vi "map.get.vi"(11 "CLZ Comics in":refnum<class "CLZ Comics.lvclass">) -> (2 "map":map{i32, T1}(c390), 3 "CLZ Comics out":refnum<class "CLZ Comics.lvclass">)   [LabVIEW 2024, in "CLZ_to_ComicVine.lvlib" / "CLZ Comics.lvclass"]
uses:
  CLZ Comics.lvclass
  CLZ Comics.lvclass/CLZ Comics.ctl
  typedefs/issue_number--cluster.ctl
  typedefs/volume--cluster.ctl
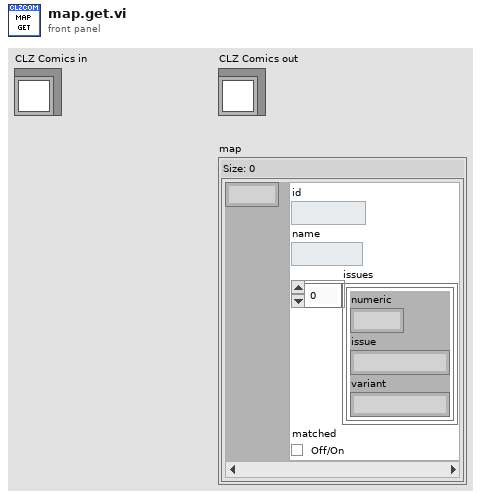
[diagram p1: front panel]
types:
  T1 = typedef "CLZ_to_ComicVine.lvlib/CLZ Comics.lvclass/volume--cluster.ctl" = cluster{"id":i32, "name":string, "issues":T2[], "matched":bool}
  T2 = typedef "CLZ_to_ComicVine.lvlib/CLZ Comics.lvclass/issue_number--cluster.ctl" = cluster{"numeric":dbl, "issue":string, "variant":string}
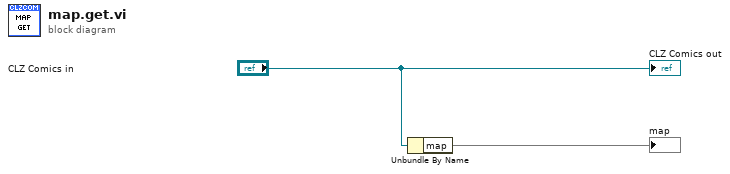
[diagram p0: block diagram]
diagram:
  n1 = Unbundle By Name("CLZ Comics in") -> ("map"=→"map":map{i32, T1})
  "CLZ Comics out" <- "CLZ Comics in"
